vi "StahlPS_Pbus.UpdateRegulation.vi"(0 "i ref in":refnum<vi>, 1 "badValue":bool, 2 "moduleValue":dbl format="%.2f", 3 "ms timeout (10000)":i32=10000, 4 "voltageRegulation":bool, 5 "error in (no error)":errorcluster, 6 "valueQuality":i32) -> (14 "i ref out":refnum<vi>, 17 "timed out":bool, 19 "error out":errorcluster)   [LabVIEW 2014, in "StahlPS_Pbus.lvlib"]
doc: "Takes the value published by the module and calculates the on-off state.\n\nThe value is written to the attribute data and published via DIM.\n\nThe bad-status bit is also determined and updated."
uses:
  StahlPS_Pbus.lvlib
  CSCore/CSApplicationBaseClasses/PSChannelBase/PSChannelBase.statusType.ctl
  CSCore/CSApplicationBaseClasses/PSChannelBase/PSChannelBase.directionType.ctl
  CSCore/CSApplicationBaseClasses/PSChannelBase/PSChannelBase.serviceType.ctl
  CSCore/CSApplicationBaseClasses/PSChannelBase/PSChannelBase.lvlib
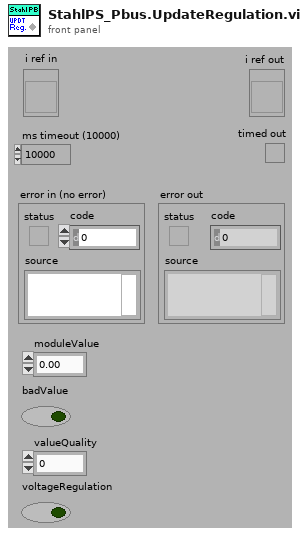
[diagram p1: front panel]
types:
  T1 = typedef "PSChannelBase.lvlib/PSChannelBase.statusType.ctl" = i32
  T2 = typedef "PSChannelBase.lvlib/PSChannelBase.serviceType.ctl" = enum16{"onOff", "voltage", "current", "tripCurrent", "rampUpSpeed", "rampDownSpeed", "status"}
  T3 = typedef "PSChannelBase.lvlib/PSChannelBase.directionType.ctl" = enum16{"unknown", "update actual value", "update nominal value", "update both"}
  T4 = typedef "StahlPS_Pbus.lvlib/StahlPS_Pbus.i attribute.ctl" = cluster{"Type":string, "CALC_FACTOR_SET_VOLTAGE":dbl, "CALC_FACTOR_GET_VOLTAGE":dbl, "CALC_FACTOR_GET_CURRENT":dbl, "CALC_FACTOR_SET_CURRENT ":dbl, "REG_VALUE":dbl, "Sign":bool, "setVoltIDs":i32[], "Elektrode Names":string[]}
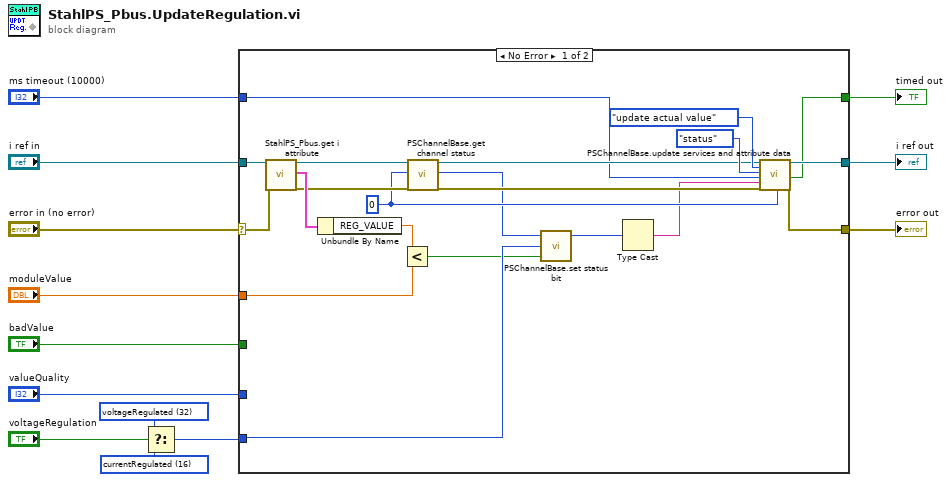
[diagram p0: block diagram]
diagram:
  w1 = T1 32 items=["onOff"=1, "inRange"=2, "rampingUp"=4, "rampingDown"=8, "currentRegulated"=16, "voltageRegulated"=32, "reserved1"=64, "reserved2"=128, "reserved3"=256, "reserved4"=512, "reserved5"=1024, "reserved6"=2048, "reserved7"=4096, "reserved8"=8192, "reserved9"=16384, "reserved10"=32768, "reserved11"=65536, "user1"=131072, "user2"=262144, "user3"=524288, "user4"=1048576, "user5"=2097152, "user6"=4194304, "user7"=8388608, "user8"=16777216, "user9"=33554432, "user10"=67108864, "user11"=134217728, "tripped"=268435456, "warning"=536870912, "error"=1073741824] ("t")
  w6 = T1 16 items=["onOff"=1, "inRange"=2, "rampingUp"=4, "rampingDown"=8, "currentRegulated"=16, "voltageRegulated"=32, "reserved1"=64, "reserved2"=128, "reserved3"=256, "reserved4"=512, "reserved5"=1024, "reserved6"=2048, "reserved7"=4096, "reserved8"=8192, "reserved9"=16384, "reserved10"=32768, "reserved11"=65536, "user1"=131072, "user2"=262144, "user3"=524288, "user4"=1048576, "user5"=2097152, "user6"=4194304, "user7"=8388608, "user8"=16777216, "user9"=33554432, "user10"=67108864, "user11"=134217728, "tripped"=268435456, "warning"=536870912, "error"=1073741824] ("f")
  n1 = Select(t=w1, s="voltageRegulation", f=w6) -> (s? t:f=w5:T1)
  n2 = case shown="No Error" "error in (no error)" {
    selector: "error in (no error)" -> [w33 w35]
    tunnel: [w28 w35] -> w10
    tunnel: "i ref in" -> [w34 w36]
    tunnel: [w29 w36] -> w9
    tunnel: "moduleValue" -> [w30 _]
    tunnel: "ms timeout (10000)" -> [w19 _]
    tunnel: [w18 _] -> w8
    tunnel: w5 -> [w15 _]
    tunnel: "valueQuality" -> [_ _]
    tunnel: "badValue" -> [_ _]
    frame No Error {
      w21 = 0 ("channelNumber")
      n3 = call "StahlPS_Pbus.get i attribute.vi"("i ref in"=w34, "error in (no error)"=w33) -> ("i ref out"=w25:refnum<vi>, "i attribute"=w32:T4, "error out"=w24:errorcluster)  [unwired: 15 in]
      n4 = Unbundle By Name(w32) -> ("REG_VALUE"=w31:dbl)
      n5 = Less?(x=w31, y=w30) -> (x < y?=w14:bool)
      n6 = call "PSChannelBase.get channel status.vi"("i ref in"=w25, "channelIndex"=w21, "error in (no error)"=w24) -> ("i ref out"=w22:refnum<vi>, "status"=w17:i32, "error out"=w23:errorcluster)  [unwired: 14 in]
      n7 = call "PSChannelBase.set status bit.vi"("set"=w14, "statusBit"=w15, "status"=w17) -> ("status out"=w16:T1)  [unwired: 2 in]
      n8 = Type Cast(x=w16) -> (*(type *) &x=w20:string)  [unwired: 1 in]
      n9 = call "PSChannelBase.update services and attribute data.vi"("i ref in"=w22, "direction"=PSChannelBase.directionType."update actual value", "service"=PSChannelBase.serviceType."status", "ms timeout (10000)"=w19, "value"=w20, "error in (no error)"=w23, "channelNumber"=w21) -> ("i ref out"=w29:refnum<vi>, "timed out"=w18:bool, "error out"=w28:errorcluster)  [unwired: 10 in]
    }
    frame Error {
    }
  }
  "error out" <- w10
  "i ref out" <- w9
  "timed out" <- w8
